vi "Setup Model.vi"(8 "error in (no error)":errorcluster, 9 "User Events in":refnum<class "User Events.lvclass">, 11 "Boot Loader in":refnum<class "Boot Loader.lvclass">) -> (0 "error out":errorcluster, 1 "User Events out":refnum<class "User Events.lvclass">, 2 "Model out":refnum<class "Model.lvclass">, 3 "Boot Loader out":refnum<class "Boot Loader.lvclass">)   [LabVIEW 2015, in "Boot Loader.lvclass"]
uses:
  Boot Loader.lvclass
  Model/Model.lvclass
  User Events/User Events.lvclass
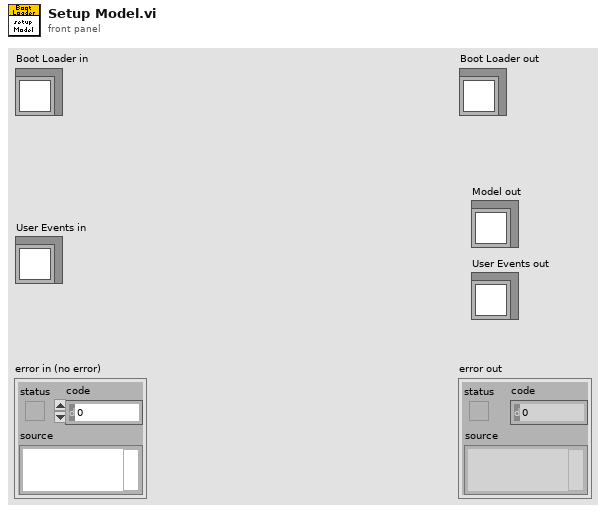
[diagram p1: front panel]
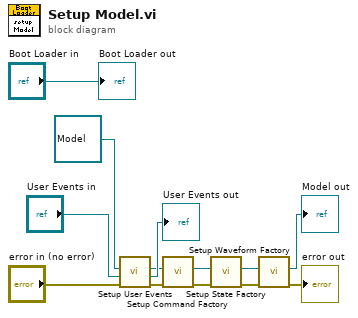
[diagram p0: block diagram]
diagram:
  n1 = call "Setup User Events.vi"("error in (no error)"="error in (no error)", "User Events in"="User Events in", "Model in"=refnum<class "Model.lvclass"> refnum) -> ("error out"=w6:errorcluster, "User Events out"=→"User Events out":refnum<class "User Events.lvclass">, "Model out"=w10:refnum<class "Model.lvclass">)  [unwired: 5 in, 1 out]
  n2 = call "Setup Command Factory.vi"("error in (no error)"=w6, "Model in"=w10) -> ("error out"=w5:errorcluster, "Model out"=w9:refnum<class "Model.lvclass">)  [unwired: 7 in, 1 out]
  n3 = call "Setup State Factory.vi"("error in (no error)"=w5, "Model in"=w9) -> ("error out"=w4:errorcluster, "Model out"=w7:refnum<class "Model.lvclass">)  [unwired: 7 in, 1 out]
  n4 = call "Setup Waveform Factory.vi"("error in (no error)"=w4, "Model in"=w7) -> ("error out"=→"error out":errorcluster, "Model out"=→"Model out":refnum<class "Model.lvclass">)  [unwired: 7 in, 1 out]
  "Boot Loader out" <- "Boot Loader in"
